vi "Load Custom Waveform.vi"(11 "Suggested Sample Rate":dbl) -> (2 "Waveform Created?":bool, 3 "Output Waveform":waveform(dbl))   [LabVIEW 2025, in "TDMS Waveform Creator UI.lvlib"]
uses:
  TDMS Waveform Creator UI.lvlib
panel:
  out "File Path":path
  in  "Scale":dbl=1.0 min=0.0 format="%#_6p"
  in  "Post Delay (s)":dbl min=0.0 format="%#_6p"
  in  "Pre Delay (s)":dbl min=0.0 format="%#_6p"
  in  "File Type":enum32{"CSV", "TDMS", "TDM"}(radio)
  in  "Read From":i32 caption="Read From Row/Wfm Index" min=0
  in  "Load File":bool
  in  "Suggest Naming?":bool=TRUE
  in  "Waveform Name":string
  in  "Cancel":bool
  in  "OK":bool
  out "Actual Sample Size":i32
  out "Actual Duration (s)":dbl format="%#_6p"
  out "Waveform Preview":waveform(dbl)(graph)
  in  "Sample Rate (Hz)":dbl=10000000.0 min=0.0 format="%#_6p"
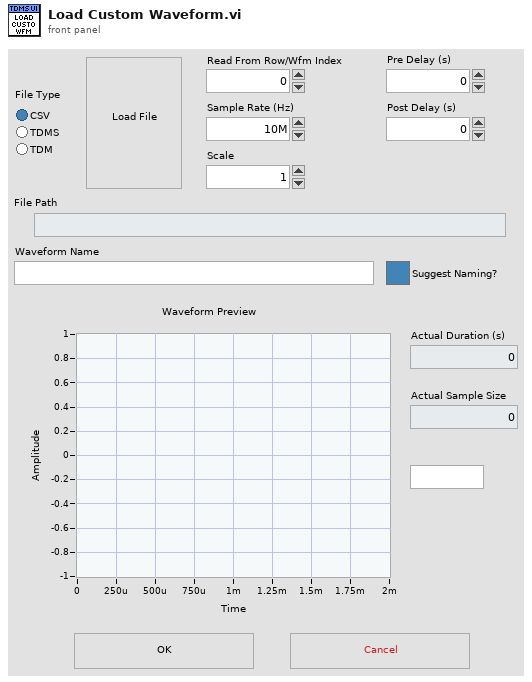
[diagram p1: front panel]
types:
  T1 = cluster{"pattern (all files)":string, "pattern label":string, "prompt":string}
  T2 = cluster{"pattern (all files)":string, "pattern label":string, "prompt":string}[]
  T3 = enum8{"Enabled", "Disabled", "Disabled and Grayed Out"}
  T4 = cluster{"File Path":string, "Sample Rate (Hz)":dbl, "Read From":i32, "Pre Delay (s)":dbl, "Post Delay (s)":dbl, "Scale":dbl}
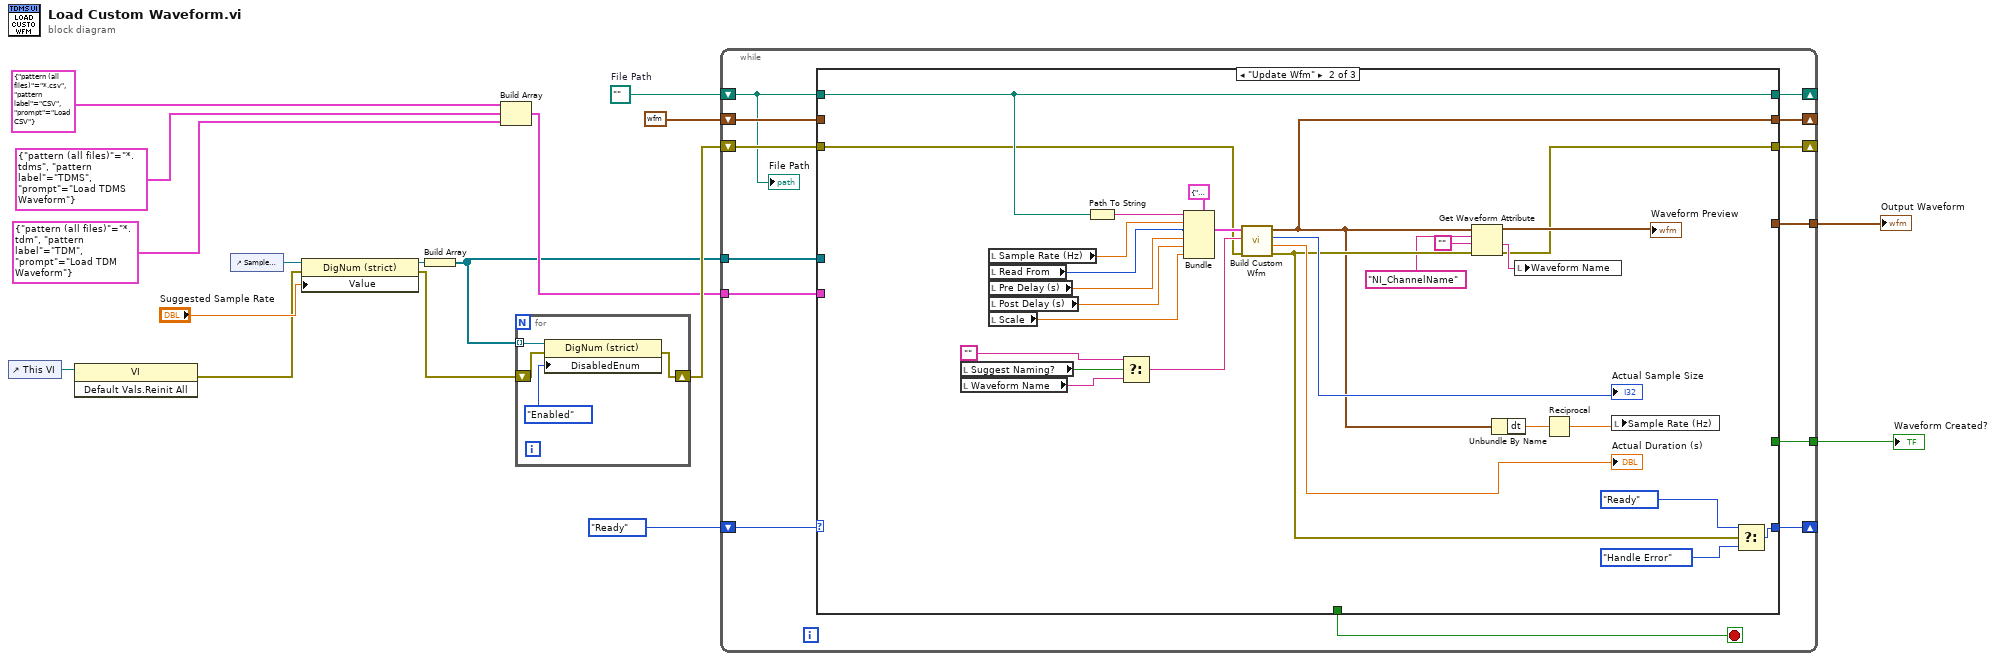
[diagram p0: block diagram]
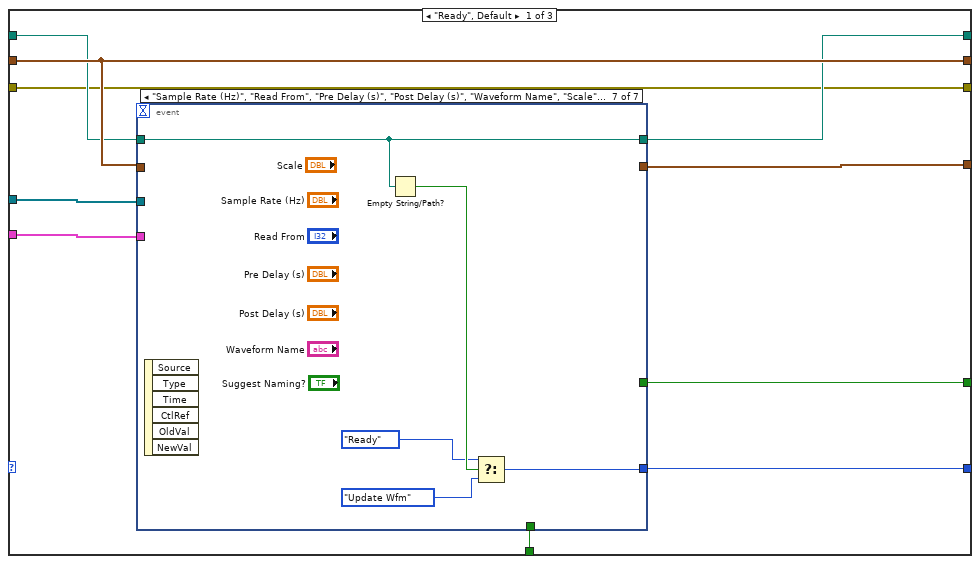
[diagram p2: hidden frame]
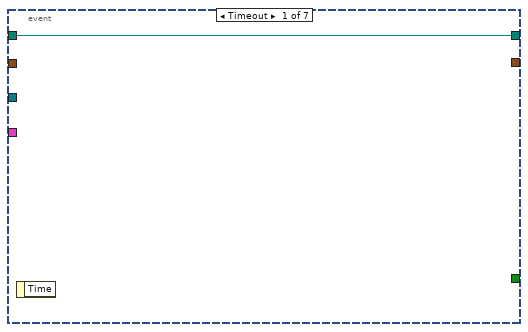
[diagram p3: hidden frame]
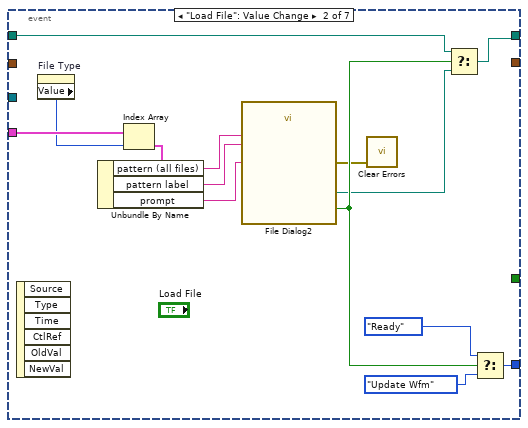
[diagram p4: hidden frame]
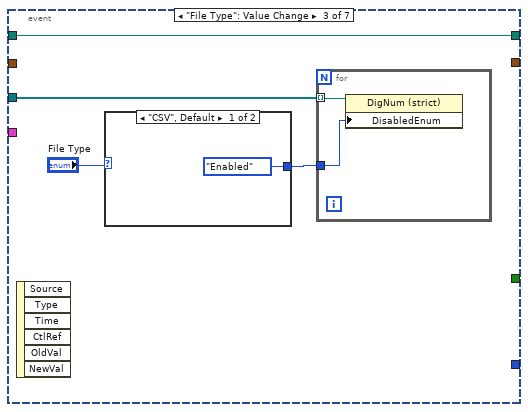
[diagram p5: hidden frame]
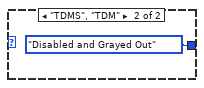
[diagram p6: hidden frame]
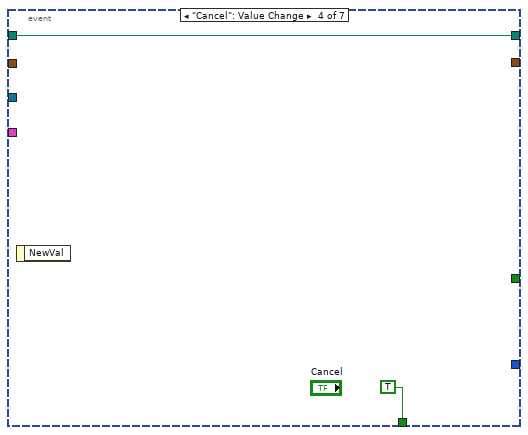
[diagram p7: hidden frame]
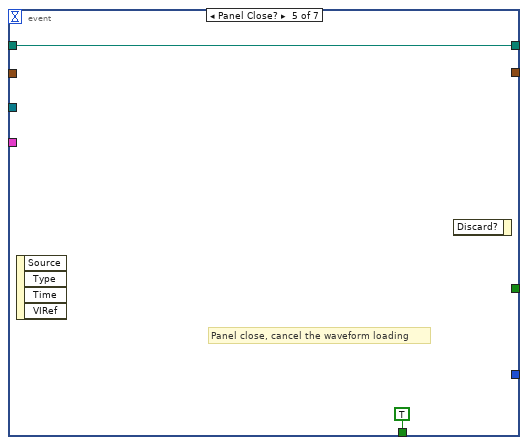
[diagram p8: hidden frame]
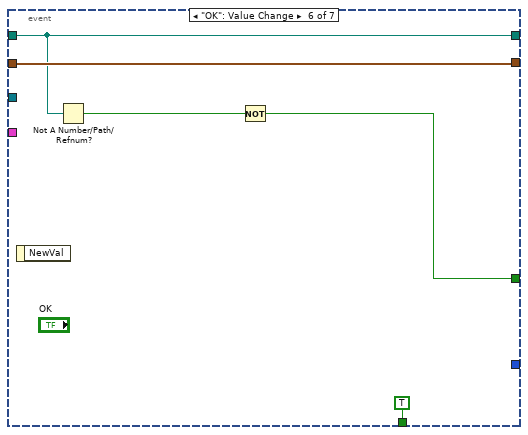
[diagram p9: hidden frame]
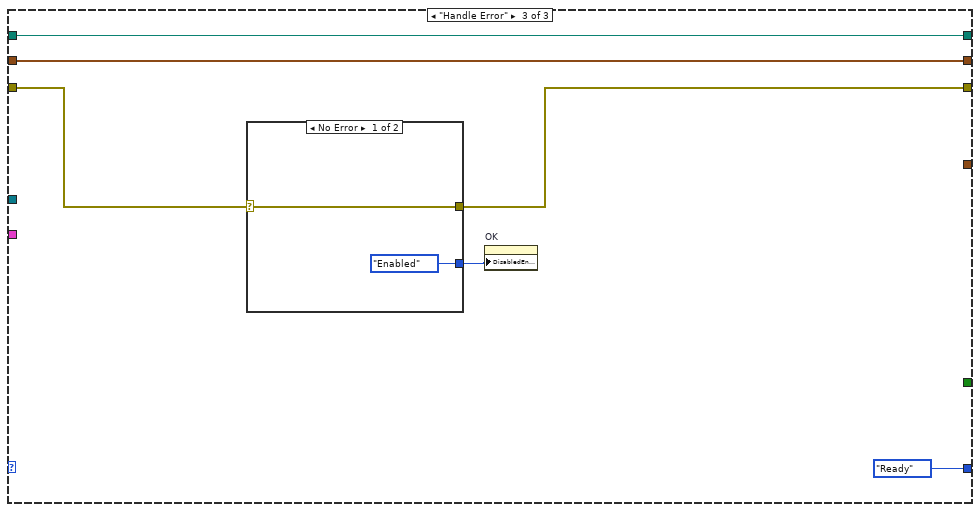
[diagram p10: hidden frame]
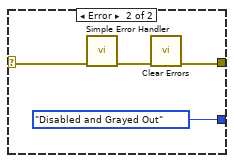
[diagram p11: hidden frame]
diagram:
  w15 = path ""  # File Path
  n1 = control-ref of="This VI"() -> (w12:refnum<vi>)
  n2 = invoke class="VI" method="Default Vals.Reinit All"(reference=w12) -> (error out=w2:errorcluster)  [unwired: 2 in, 2 out]
  n3 = control-ref of="Sample Rate (Hz)"() -> (w11:refnum<vi>)
  n4 = property class="DigNum (strict)"(reference=w11, error in=w2, "Value"="Suggested Sample Rate") -> (reference out=w4:refnum<vi>, error out=w1:errorcluster)
  n5 = Build Array(w4) -> (w6:refnum<vi>[])
  n6 = Build Array(T1 {"pattern (all files)"="*.csv", "pattern label"="CSV", "prompt"="Load CSV"}, T1 {"pattern (all files)"="*.tdms", "pattern label"="TDMS", "prompt"="Load TDMS Waveform"}, T1 {"pattern (all files)"="*.tdm", "pattern label"="TDM", "prompt"="Load TDM Waveform"}) -> (w7:T2)
  n7 = for {
    tunnel: w6 -> [w21] mode=indexing
    shift-right: [w18] -> w10
    shift-left: w1 -> [w19]
    n8 = property class="DigNum (strict)"(reference=w21, error in=w19, "DisabledEnum"=T3."Enabled" ("Disabled")) -> (error out=w18:errorcluster)  [unwired: 1 out]
  }
  n9 = while {
    tunnel: [w33] -> w17
    shift-right: [w31] -> _
    shift-left: enum16{"Ready", "Update Wfm", "Handle Error"}."Ready" -> [w32]
    shift-right: [w30] -> _
    shift-left: w15 -> [w22]
    shift-right: [w28] -> _
    shift-left: waveform(dbl) {"t0"=timestamp(0 s since 1904-01-01), "dt"=1.0, "Y"=[]} ("Output Waveform") -> [w29]
    tunnel: [w27] -> w13
    tunnel: w7 -> [w26]
    tunnel: w6 -> [w25]
    shift-right: [w23] -> _
    shift-left: w10 -> [w24]
    stop <- w34 stop-if-true
    n10 = case shown="\"Update Wfm\"" w32 {
      tunnel: [w44 _ _] -> w34
      tunnel: [w43 _ _] -> w33
      tunnel: [w42 w109 enum16{"Ready", "Update Wfm", "Handle Error"}."Ready"] -> w31
      tunnel: w22 -> [w39 w107 w114]
      tunnel: [w38 w107 w114] -> w30
      tunnel: w29 -> [w41 _ w115]
      tunnel: [w41 w88 w115] -> w28
      tunnel: [w40 _ _] -> w27
      tunnel: w26 -> [w37 _ _]
      tunnel: w25 -> [w36 _ _]
      tunnel: w24 -> [w35 w91 w112]
      tunnel: [w35 w92 w111] -> w23
      frame "Ready", Default {
        n11 = event shown="[6] \"Sample Rate (Hz)\", \"Read From\", \"Pre Delay (s)\", \"Post Delay (s)\", \"Waveform Name\", \"Scale\", \"Suggest Naming?\": Value Change" {
          selector: _ -> [_ _ _ _ _ _ _]
          dyn-events: _ -> [_ _ _ _ _ _ _]
          timeout: _ -> [_ _ _ _ _ _ _]
          tunnel: [_ _ _ TRUE TRUE TRUE _] -> w44
          tunnel: [_ _ _ _ _ w72 _] -> w43
          tunnel: [_ w59 _ _ _ _ w81] -> w42
          tunnel: w41 -> [_ _ _ _ _ w75 _]
          tunnel: [_ _ _ _ _ w75 _] -> w40
          tunnel: w39 -> [w45 w57 w63 w68 w71 w74 w80]
          tunnel: [w45 w55 w63 w68 w71 w74 w80] -> w38
          tunnel: w37 -> [_ w54 _ _ _ _ _]
          tunnel: w36 -> [_ _ w62 _ _ _ _]
          event Timeout {
            n12 = event-data() -> ()  [unwired: 1 in, 1 out]
          }
          event "Load File": Value Change {
            n13 = event-data() -> ()  [unwired: 1 in, 6 out]
            n14 = property on="File Type" class="RadioBtnsControl (strict)"() -> ("Value"=w49:enum32{"CSV", "TDMS", "TDM"})  [unwired: 2 in, 2 out]
            n15 = Index Array(array=w54, index=w49) -> (element=w53:T1)
            n16 = Unbundle By Name(w53) -> ("pattern (all files)"=w52:string, "pattern label"=w51:string, "prompt"=w50:string)
            n17 = call "File Dialog2"("prompt"=w50, "pattern (all files)"=w52, "pattern label"=w51) -> ("selected path"=w56:path, "cancelled"=w58:bool, "error out"=w48:errorcluster)  [unwired: 9 in, 1 out]
            n18 = call <vilib>:"Clear Errors.vi"("error in (no error)"=w48) -> ()  [unwired: 5 in, 2 out]
            n19 = Select(t=w57, s=w58, f=w56) -> (s? t:f=w55:path)
            n20 = Select(t=enum16{"Ready", "Update Wfm", "Handle Error"}."Ready", s=w58, f=enum16{"Ready", "Update Wfm", "Handle Error"}."Update Wfm") -> (s? t:f=w59:enum16{"Ready", "Update Wfm", "Handle Error"})
          }
          event "File Type": Value Change {
            n21 = event-data() -> ()  [unwired: 1 in, 6 out]
            n22 = case shown="\"CSV\", Default" "File Type" {
              tunnel: [T3."Enabled" ("Disabled") T3."Disabled and Grayed Out" ("Disabled")] -> w61
              frame "CSV", Default {
              }
              frame "TDMS", "TDM" {
              }
            }
            n23 = for {
              tunnel: w62 -> [w67] mode=indexing
              tunnel: w61 -> [w66]
              n24 = property class="DigNum (strict)"(reference=w67, "DisabledEnum"=w66) -> ()  [unwired: 1 in, 2 out]
            }
          }
          event "Cancel": Value Change {
            n25 = event-data() -> ()  [unwired: 1 in, 1 out]
          }
          event Panel Close? {
            # "Panel close, cancel the waveform loading"
            n26 = event-data() -> ()  [unwired: 1 in, 4 out]
            n27 = event-data() -> ()  [unwired: 2 in, 1 out]
          }
          event "OK": Value Change {
            n28 = event-data() -> ()  [unwired: 1 in, 1 out]
            n29 = Not A Number/Path/Refnum?(number/path/refnum=w74) -> (NaN/Path/Refnum?=w73:bool)
            n30 = Not(x=w73) -> (.not. x?=w72:bool)
          }
          event "Sample Rate (Hz)", "Read From", "Pre Delay (s)", "Post Delay (s)", "Waveform Name", "Scale", "Suggest Naming?": Value Change {
            n31 = event-data() -> ()  [unwired: 1 in, 6 out]
            n32 = Empty String/Path?(string/path=w80) -> (empty?=w79:bool)
            n33 = Select(t=enum16{"Ready", "Update Wfm", "Handle Error"}."Ready", s=w79, f=enum16{"Ready", "Update Wfm", "Handle Error"}."Update Wfm") -> (s? t:f=w81:enum16{"Ready", "Update Wfm", "Handle Error"})
          }
        }
      }
      frame "Update Wfm" {
        n34 = local read "Suggest Naming?"() -> (w97:bool)
        n35 = local read "Waveform Name"() -> (w93:string)
        n36 = local read "Sample Rate (Hz)"() -> (w106:dbl)
        n37 = local read "Read From"() -> (w105:i32)
        n38 = local read "Pre Delay (s)"() -> (w84:dbl)
        n39 = local read "Post Delay (s)"() -> (w104:dbl)
        n40 = local read "Scale"() -> (w82:dbl)
        n41 = Path To String(path=w107) -> (string=w85:string)
        n42 = Select(t="", s=w97, f=w93) -> (s? t:f=w103:string)
        n43 = Bundle(cluster=T4 {"File Path"="", "Sample Rate (Hz)"=10000000.0, "Read From"=0, "Pre Delay (s)"=0.0, "Post Delay (s)"=0.0, "Scale"=1.0} ("Custom Wfm Config"), "File Path"=w85, "Sample Rate (Hz)"=w106, "Read From"=w105, "Pre Delay (s)"=w84, "Post Delay (s)"=w104, "Scale"=w82) -> (w108:T4)
        n44 = call "Build Custom Wfm.vi"("error in"=w91, "User Provided Name"=w103, "Custom Wfm Config"=w108) -> ("error out"=w99:errorcluster, "Actual Duration (s)"=→"Actual Duration (s)":dbl, "Actual Sample Size"=→"Actual Sample Size":i32, "Waveform"=w88:waveform(dbl))  [unwired: 5 in]
        n45 = Get Waveform Attribute(4:w99, 5:"", 6:"NI_ChannelName" ("name"), 7:w88) -> (0:w92:errorcluster, 1:w94:string, 3:→"Waveform Preview":waveform(dbl))  [unwired: 1 out]
        n46 = Unbundle By Name(w88) -> ("dt"=w87:dbl)
        n47 = local write "Waveform Name"(w94) -> ()
        n48 = Reciprocal(x=w87) -> (1/x=w86:dbl)
        n49 = local write "Sample Rate (Hz)"(w86) -> ()
        n50 = Select(t=enum16{"Ready", "Update Wfm", "Handle Error"}."Ready", s=w99, f=enum16{"Ready", "Update Wfm", "Handle Error"}."Handle Error") -> (s? t:f=w109:enum16{"Ready", "Update Wfm", "Handle Error"})
      }
      frame "Handle Error" {
        n51 = case shown="No Error" w112 {
          selector: w112 -> [w117 w121]
          tunnel: [w117 w118] -> w111
          tunnel: [T3."Enabled" ("DisabledEnum") T3."Disabled and Grayed Out" ("DisabledEnum")] -> w113
          frame No Error {
          }
          frame Error {
            n52 = call <vilib>:"Simple Error Handler.vi"("error in (no error)"=w121) -> ("error out"=w120:errorcluster)  [unwired: 4 in, 4 out]
            n53 = call <vilib>:"Clear Errors.vi"("error in (no error)"=w120) -> ("error out"=w118:errorcluster)  [unwired: 5 in, 1 out]
          }
        }
        n54 = property on="OK" class="Bool"("DisabledEnum"=w113) -> ()  [unwired: 2 in, 2 out]
      }
    }
    "File Path" <- w22
  }
  "Waveform Created?" <- w17
  "Output Waveform" <- w13
